vi "Update CPU UI Components.vi"(8 "error in (no error)":errorcluster, 10 "CPU Metrics":T1, 11 "Application Manager in":refnum<class "Application Manager.lvclass">) -> (0 "error out":errorcluster, 3 "Application Manager out":refnum<class "Application Manager.lvclass">)   [LabVIEW 2020, in "Application Manager.lvlib" / "Application Manager.lvclass"]
uses:
  Application Manager.lvclass
  CPU FFT Calculator/CPU FFT Calculator/CPU Metrics.ctl
  Application Manager.lvclass/Application Manager.ctl
  Simple UI/Simple UI/Simple UI.lvclass
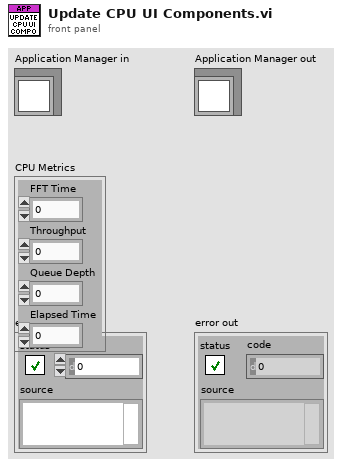
[diagram p1: front panel]
types:
  T1 = typedef "Simple UI.lvlib/Simple UI.lvclass/CPU Metrics.ctl" = cluster{"FFT Time":dbl, "Throughput":dbl, "Queue Depth":u64, "Elapsed Time":dbl}
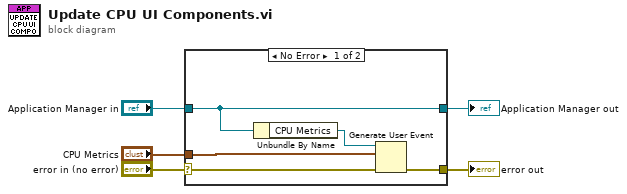
[diagram p0: block diagram]
diagram:
  n1 = case shown="No Error" "error in (no error)" {
    selector: "error in (no error)" -> [w7 w12]
    tunnel: [w6 w12] -> w4
    tunnel: [w10 w11] -> w2
    tunnel: "Application Manager in" -> [w10 w11]
    tunnel: "CPU Metrics" -> [w8 _]
    frame No Error {
      n2 = Unbundle By Name(w10) -> ("CPU Metrics"=w9:refnum<user-event>)
      n3 = Generate User Event(user event=w9, event data cluster=w8, error in=w7) -> (error out=w6:errorcluster)  [unwired: 1 in, 1 out]
    }
    frame Error {
    }
  }
  "error out" <- w4
  "Application Manager out" <- w2
